vi "Analog Trigger with Interleaving Select.vi"(0 "all channels":cluster{fxp<+/-,12,1>[]}[](array[cluster])=[{[0.0, 0.0, 0.0, 0.0, 0.0, 0.0, 0.0, 0.0, 0.0, 0.0, 0.0, 0.0, 0.0, 0.0, 0.0, 0.0]}, {[0.0, 0.0, 0.0, 0.0, 0.0, 0.0, 0.0, 0.0, 0.0, 0.0, 0.0, 0.0, 0.0, 0.0, 0.0, 0.0]}], 1 "interleaving factor":u16, 5 "channel":fxp<+,2,2> format="%#_4g", 7 "trigger level":fxp<+/-,32,1>, 9 "hysteresis level":fxp<+/-,32,1>, 11 "rising edge":bool=TRUE) -> (6 "triggered":bool)   [LabVIEW 2018, in "GettingStarted_5775_FPGA.lvlib"]
uses:
  GettingStarted_5775_FPGA.lvlib
  db24aacc-3aa9-45e6-b75f-233848c1dcdd.vi
  1961724d-2c00-4db4-be5f-47e2776cd38e.vi
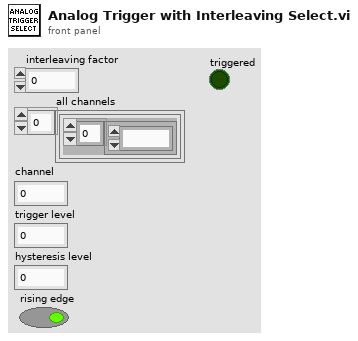
[diagram p1: front panel]
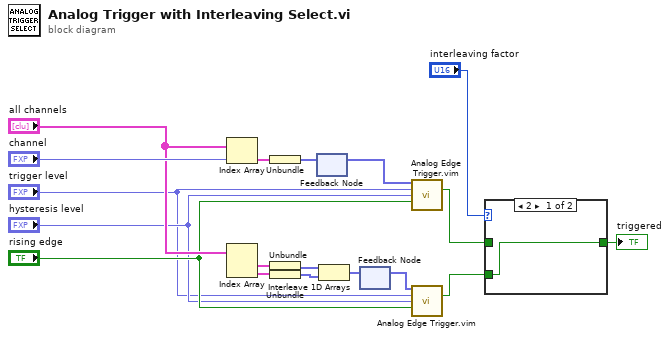
[diagram p0: block diagram]
diagram:
  n1 = Index Array(array="all channels", index="channel") -> (element=w10:cluster{fxp<+/-,12,1>[]})
  n2 = Index Array(array="all channels") -> (element #1=w13:cluster{fxp<+/-,12,1>[]}, element #2=w14:cluster{fxp<+/-,12,1>[]})  [unwired: 2 in]
  n3 = Unbundle(w10) -> (w11:fxp<+/-,12,1>[])
  n4 = Unbundle(w13) -> (w15:fxp<+/-,12,1>[])
  n5 = Unbundle(w14) -> (w16:fxp<+/-,12,1>[])
  n6 = feedback #1() -> (w9:fxp<+/-,12,1>[])  [unwired: 1 in]
  n7 = feedback-in #1(w11) -> ()
  n8 = Interleave 1D Arrays(w15, w16) -> (w17:fxp<+/-,12,1>[])
  n9 = feedback #2() -> (w12:fxp<+/-,12,1>[])  [unwired: 1 in]
  n10 = feedback-in #2(w17) -> ()
  n11 = call "Analog Edge Trigger.vim"("trigger channel data"=w9, "requested trigger level"="trigger level", "requested hysteresis level"="hysteresis level", "rising edge"="rising edge") -> ("triggered"=w2:bool)  [unwired: 8 in, 3 out]
  n12 = call "Analog Edge Trigger.vim"("trigger channel data"=w12, "requested trigger level"="trigger level", "requested hysteresis level"="hysteresis level", "rising edge"="rising edge") -> ("triggered"=w3:bool)  [unwired: 8 in, 3 out]
  n13 = case shown="2" "interleaving factor" {
    tunnel: w3 -> [w19 _]
    tunnel: [w19 w20] -> w1
    tunnel: w2 -> [_ w20]
    frame 2 {
    }
    frame 1, Default {
    }
  }
  "triggered" <- w1
